vi "Corr Digitizer Open.vi"(8 "error in":errorcluster, 11 "digitizer corrections in":T1) -> (0 "error out":errorcluster, 1 "all channels of the correction valid?":bool, 2 "some correction selected?":bool, 3 "digitizer corrections out":T1)   [LabVIEW 2013]
doc: "This VI will invoke open dialog for digitizer correction selection. If selected it will load it and check if it is valid."
uses:
  Corr Digitizers.ctl
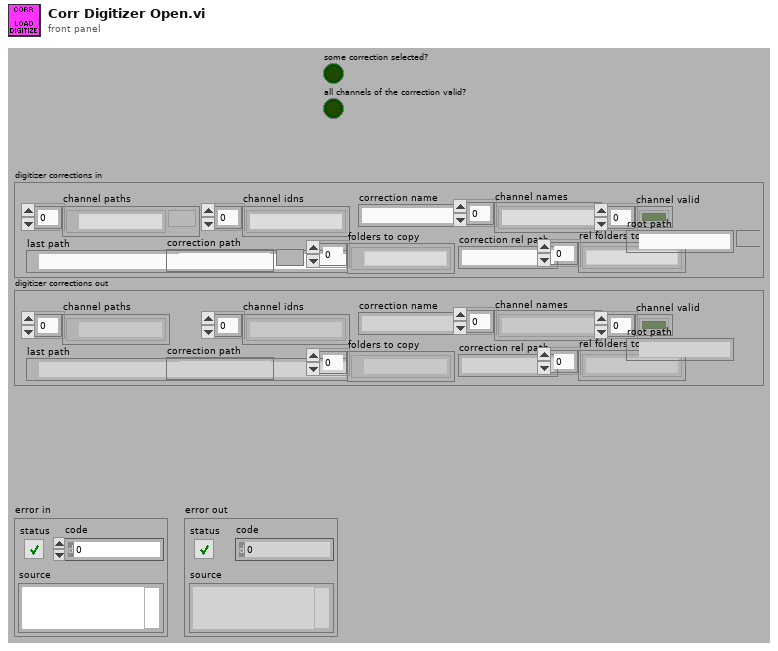
[diagram p1: front panel]
types:
  T1 = typedef "Corr Digitizers.ctl" = cluster{"last path":path, "channel paths":path[], "channel idns":string[], "correction name":string, "channel names":string[], "folders to copy":path[], "channel valid":bool[], "correction path":path, "correction rel path":string, "rel folders to copy":string[], "root path":path}
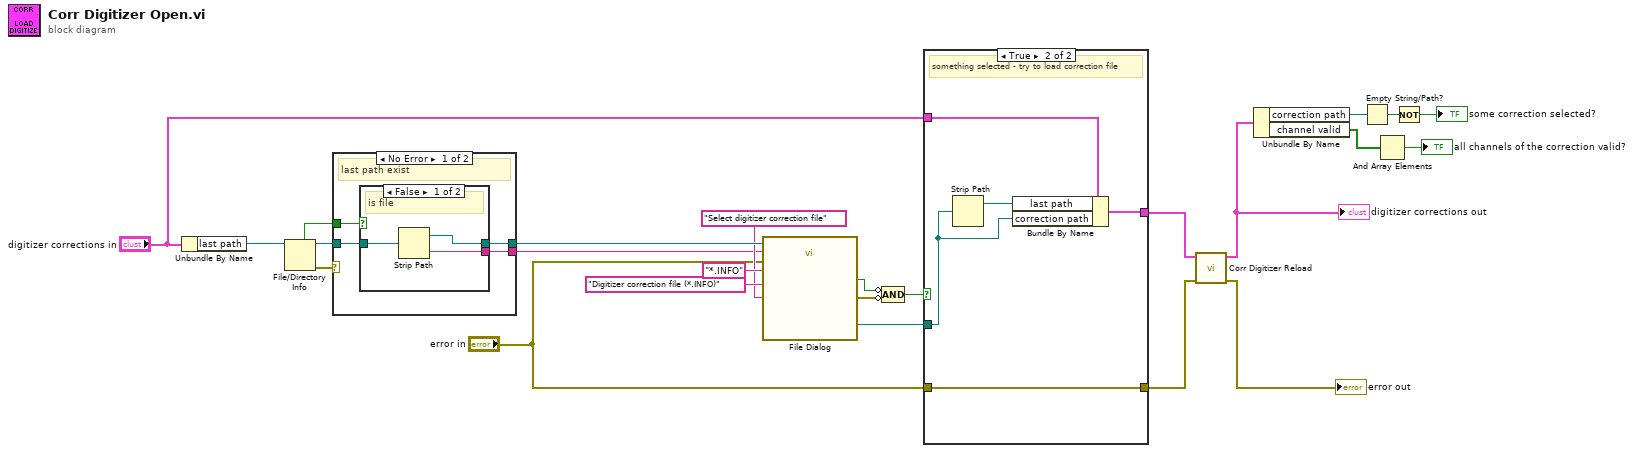
[diagram p0: block diagram]
diagram:
  n1 = Unbundle By Name("digitizer corrections in") -> ("last path"=w24:path)
  n2 = File/Directory Info(path=w24) -> (path out=w22:path, directory=w21:bool, error out=w23:errorcluster)  [unwired: 1 in, 4 out]
  n3 = case shown="No Error" w23 {
    tunnel: w22 -> [w27 w33]
    tunnel: w21 -> [w28 _]
    tunnel: [w26 w33] -> w20
    tunnel: [w25 _] -> w1
    frame No Error {
      # "last path exist"
      n4 = case shown="False" w28 {
        tunnel: w27 -> [w31 w32]
        tunnel: [w30 w32] -> w26
        tunnel: [w29 _] -> w25
        frame False {
          # "is file"
          n5 = Strip Path(path=w31) -> (stripped path=w30:path, name=w29:string)
        }
        frame True {
          # "is folder"
        }
      }
    }
    frame Error {
    }
  }
  n6 = call "File Dialog"("start path"=w20, "prompt"="Select digitizer correction file", "default name"=w1, "error in"="error in", "pattern (all files)"="*.INFO", "pattern label"="Digitizer correction file (*.INFO)") -> ("selected path"=w13:path, "cancelled"=w16:bool, "error out"=w14:errorcluster)  [unwired: 6 in, 1 out]
  n7 = Compound Arithmetic op=AND(invert w16, invert w14) -> (w15:bool)
  n8 = case shown="True" w15 {
    tunnel: w13 -> [_ w38]
    tunnel: "error in" -> [w35 w37]
    tunnel: [w35 w37] -> w9
    tunnel: "digitizer corrections in" -> [w34 w40]
    tunnel: [w34 w36] -> w10
    frame False {
    }
    frame True {
      # "something selected - try to load correction file"
      n9 = Strip Path(path=w38) -> (stripped path=w39:path)  [unwired: 1 out]
      n10 = Bundle By Name(cluster=w40, "last path"=w39, "correction path"=w38) -> (w36:T1)
    }
  }
  n11 = call "Corr Digitizer Reload.vi"("error in (no error)"=w9, "digitizer corrections in"=w10) -> ("error out"=→"error out":errorcluster, "digitizer corrections out"=w7:T1)  [unwired: 8 in]
  "digitizer corrections out" <- w7
  n12 = Unbundle By Name(w7) -> ("correction path"=w6:path, "channel valid"=w5:bool[])
  n13 = Empty String/Path?(string/path=w6) -> (empty?=w4:bool)
  n14 = And Array Elements(Boolean array=w5) -> (logical AND=→"all channels of the correction valid?":bool)
  n15 = Not(x=w4) -> (.not. x?=→"some correction selected?":bool)
